vi "BL_IsChannelPlugged.vi"(8 "error in (no error)":errorcluster, 10 "Channel":u8 max=15, 11 "Potentiostat Galvanostat in":refnum<class "Potentiostat Galvanostat.lvclass">) -> (0 "error out":errorcluster, 1 "Is Channel Plugged?":bool, 2 "Channel":u8, 3 "Potentiostat Galvanostat out":refnum<class "Potentiostat Galvanostat.lvclass">)   [LabVIEW 2018, in "Potentiostat Galvanostat.lvclass"]
doc: "This function tests the communication speed between the library and the selected channel. \nNOTE: This function is for advanced user only."
uses:
  Potentiostat Galvanostat.lvclass
  Potentiostat Galvanostat.lvclass/Potentiostat Galvanostat.ctl
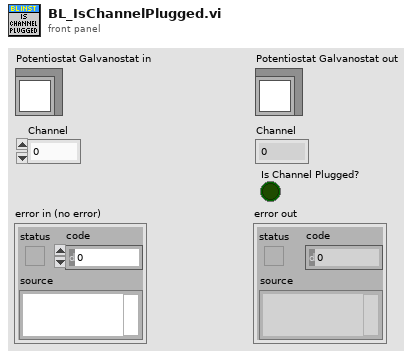
[diagram p1: front panel]
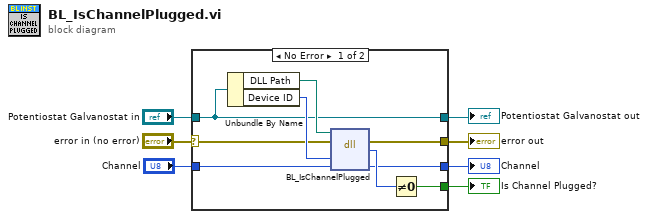
[diagram p0: block diagram]
diagram:
  n1 = case shown="No Error" "error in (no error)" {
    selector: "error in (no error)" -> [w13 w18]
    tunnel: [w12 w18] -> w6
    tunnel: [w10 w17] -> w4
    tunnel: "Potentiostat Galvanostat in" -> [w10 w17]
    tunnel: "Channel" -> [w9 _]
    tunnel: [w11 _] -> w2
    tunnel: [w8 _] -> w1
    frame No Error {
      n2 = Unbundle By Name(w10) -> ("DLL Path"=w15:path, "Device ID"=w14:i32)
      n3 = dll-call lib="C:/Program Files (x86)/National Instruments/LabVIEW 2018/user.lib/EClib/EClib.*" fn="BL_IsChannelPlugged"(path in=w15, error in=w13, "Device ID"=w14, "Channel"=w9) -> (error out=w12:errorcluster, "Is Channel Plugged?"=w16:u8, "Channel"=w8:u8)  [unwired: 2 in, 1 out]
      n4 = Not Equal To 0?(x=w16) -> (x != 0?=w11:bool)
    }
    frame Error {
    }
  }
  "error out" <- w6
  "Potentiostat Galvanostat out" <- w4
  "Is Channel Plugged?" <- w2
  "Channel" <- w1
